vi "Math-Loess Smooth.vi"(8 "Robust?":bool, 9 "Quadratic?":bool, 10 "Span":i32, 11 "Array":dbl[](array[numeric])) -> (3 "Smoothed Array":dbl[](array[numeric]))   [LabVIEW 2020]
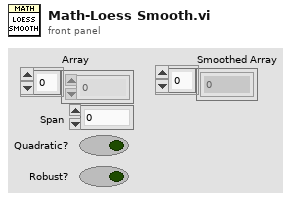
[diagram p1: front panel]
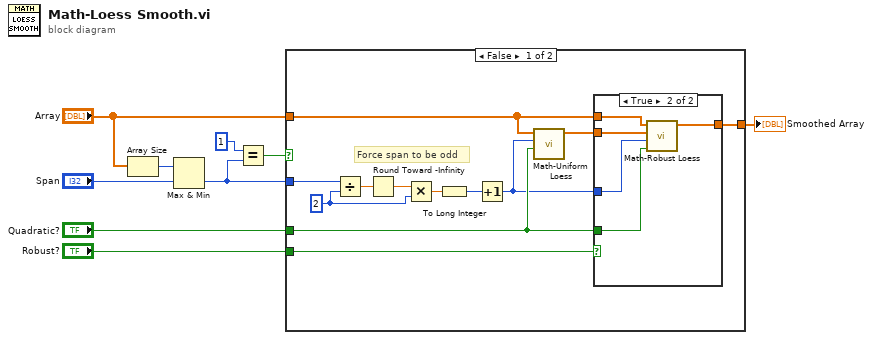
[diagram p0: block diagram]
diagram:
  n1 = Array Size(array="Array") -> (size(s)=w9:i32)
  n2 = Max & Min(x=w9, y="Span") -> (min(x,y)=w3:i32)  [unwired: 1 out]
  n3 = Equal?(x=1 ("y"), y=w3) -> (x = y?=w4:bool)
  n4 = case shown="False" w4 {
    tunnel: "Array" -> [w10 w28]
    tunnel: [w13 w28] -> w5
    tunnel: w3 -> [w21 _]
    tunnel: "Quadratic?" -> [w12 _]
    tunnel: "Robust?" -> [w15 _]
    frame False {
      w18 = 2 ("y")
      # "Force span to be odd"
      n5 = Divide(x=w21, y=w18) -> (x/y=w20:dbl)
      n6 = Round Toward -Infinity(1:w20) -> (0:w19:dbl)
      n7 = Multiply(x=w19, y=w18) -> (x*y=w17:dbl)
      n8 = To Long Integer(number=w17) -> (32bit integer=w16:i32)
      n9 = Increment(x=w16) -> (x+1=w11:i32)
      n10 = call "Math-Uniform Loess.vi"("Quadratic?"=w12, "Span"=w11, "Array"=w10) -> ("Smoothed Array"=w14:dbl[])  [unwired: 8 in]
      n11 = case shown="True" w15 {
        tunnel: w14 -> [w22 w24]
        tunnel: [w22 w27] -> w13
        tunnel: w12 -> [_ w26]
        tunnel: w11 -> [_ w25]
        tunnel: w10 -> [_ w23]
        frame False {
        }
        frame True {
          n12 = call "Math-Robust Loess.vi"("Quadratic?"=w26, "Span"=w25, "Nonrobust Smoothed"=w24, "Array"=w23) -> ("Robust Smoothed"=w27:dbl[])  [unwired: 7 in]
        }
      }
    }
    frame True {
      # "Span=1: no smoothing, return original array"
    }
  }
  "Smoothed Array" <- w5
